vi "Check for Data File Exists.vi"(2 "error in":errorcluster, 3 "File Details":cluster{"Data Path":path, "Position Number":i8}) -> (0 "error out":errorcluster, 1 "refnum Out":refnum<file>)   [LabVIEW 2021]
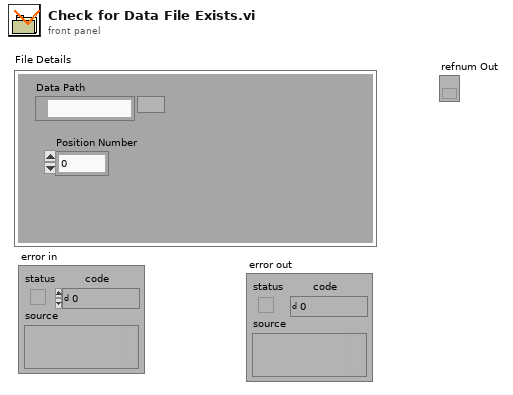
[diagram p1: front panel]
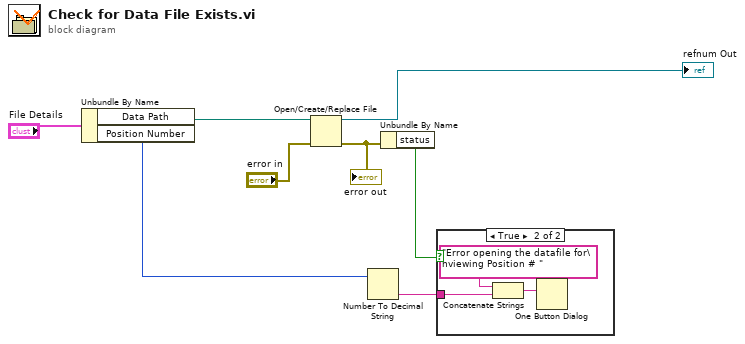
[diagram p0: block diagram]
diagram:
  n1 = Unbundle By Name("File Details") -> ("Data Path"=w4:path, "Position Number"=w2:i8)
  n2 = Open/Create/Replace File(file path (use dialog)=w4, error in="error in") -> (refnum out=→"refnum Out":refnum<file>, error out=w7:errorcluster)  [unwired: 4 in, 1 out]
  "error out" <- w7
  n3 = Number To Decimal String(number=w2) -> (decimal integer string=w5:string)  [unwired: 1 in]
  n4 = Unbundle By Name(w7) -> ("status"=w6:bool)
  n5 = case shown="True" w6 {
    tunnel: w5 -> [_ w10]
    frame False {
    }
    frame True {
      n6 = Concatenate Strings("Error opening the datafile for\nviewing Position # ", w10) -> (w9:string)
      n7 = One Button Dialog(message=w9) -> ()  [unwired: 1 in, 1 out]
    }
  }
